vi "Priority.vi"(8 "error in (no error)":errorcluster, 11 "WebSocket Handler in":refnum<class "WebSocket Handler.lvclass">) -> (0 "error out":errorcluster, 2 "Priority":u16, 3 "WebSocket Handler out":refnum<class "WebSocket Handler.lvclass">)   [LabVIEW 2020, in "HTTP Server.lvlib" / "WebSocket Handler.lvclass"]
uses:
  WebSocket Handler.lvclass
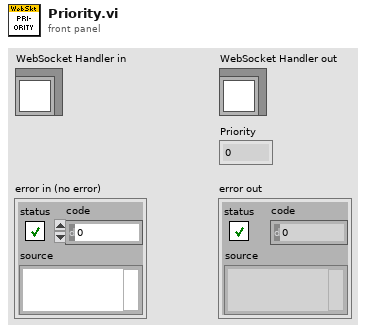
[diagram p1: front panel]
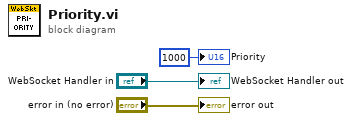
[diagram p0: block diagram]
diagram:
  "error out" <- "error in (no error)"
  "WebSocket Handler out" <- "WebSocket Handler in"
  "Priority" <- u16 1000 ("Priority")
